vi "LESO_error.vi"(8 "error in":errorcluster, 11 "FT_Status":u32(ring) items=["FT_OK", "FT_INVALID_HANDLE", "FT_DEVICE_NOT_FOUND", "FT_DEVICE_NOT_OPENED", "FT_IO_ERROR", "FT_INSUFFICIENT_RESOURCES", "FT_INVALID_PARAMETER", "FT_INVALID_BAUD_RATE", "FT_DEVICE_NOT_OPENED_FOR_ERASE", "FT_DEVICE_NOT_OPENED_FOR_WRITE", "FT_FAILED_TO_WRITE_DEVICE", "FT_EEPROM_READ_FAILED", "FT_EEPROM_WRITE_FAILED", "FT_EEPROM_ERASE_FAILED", "FT_EEPROM_NOT_PRESENT", "FT_EEPROM_NOT_PROGRAMMED", "FT_INVALID_ARGS", "FT_NOT_SUPPORTED", "FT_OTHER_ERROR"]) -> (0 "error out":errorcluster)   [LabVIEW 2012]
doc: "Преобразует <B>FT_Status</B> в ошибку. Если <B>FT_Status</B> не равен <B>FT_OK</B>, то добавляет ошибку в кластер ошибок. В описании ошибки будет имя текущего ВП и <B>FT_Status</B>."
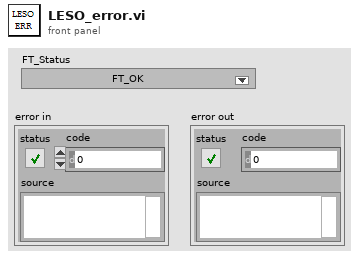
[diagram p1: front panel]
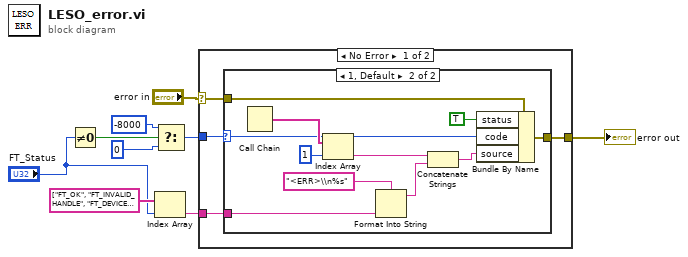
[diagram p0: block diagram]
diagram:
  n1 = Not Equal To 0?(x="FT_Status") -> (x != 0?=w8:bool)
  n2 = Index Array(array=string[] ["FT_OK", "FT_INVALID_HANDLE", "FT_DEVICE_NOT_FOUND", "FT_DEVICE_NOT_OPENED", "FT_IO_ERROR", "FT_INSUFFICIENT_RESOURCES", "FT_INVALID_PARAMETER", "FT_INVALID_BAUD_RATE", "FT_DEVICE_NOT_OPENED_FOR_ERASE", "FT_DEVICE_NOT_OPENED_FOR_WRITE", "FT_FAILED_TO_WRITE_DEVICE", "FT_EEPROM_READ_FAILED", "FT_EEPROM_WRITE_FAILED", "FT_EEPROM_ERASE_FAILED", "FT_EEPROM_NOT_PRESENT", "FT_EEPROM_NOT_PROGRAMMED", "FT_INVALID_ARGS", "FT_NOT_SUPPORTED", "FT_OTHER_ERROR"] ("Status"), index="FT_Status") -> (element=w6:string)
  n3 = Select(t=-8000 ("error code (0)"), s=w8, f=0) -> (s? t:f=w3:i32)
  n4 = case shown="No Error" "error in" {
    selector: "error in" -> [w10 w26]
    tunnel: [w13 w26] -> w2
    tunnel: w3 -> [w11 _]
    tunnel: w6 -> [w12 _]
    frame No Error {
      n5 = case shown="1, Default" w11 {
        selector: w11 -> [_ w16]
        tunnel: [w14 w25] -> w13
        tunnel: w12 -> [_ w24]
        tunnel: w10 -> [w14 w15]
        frame 0 {
          # "Статус равен нулю, ошибки нет."
        }
        frame 1, Default {
          n6 = Call Chain() -> (call chain=w21:string[])
          n7 = Index Array(array=w21, index=1) -> (element=w18:string)
          n8 = Format Into String(format string="<ERR>\\n%s", w24) -> (resulting string=w19:string)  [unwired: 2 in, 1 out]
          n9 = Concatenate Strings(w18, w19) -> (w23:string)
          n10 = Bundle By Name(cluster=w15, "status"=TRUE, "code"=w16, "source"=w23) -> (w25:errorcluster)
        }
      }
    }
    frame Error {
      # "На входе уже ошибка,\nпропускаем ее без изменений на выход"
    }
  }
  "error out" <- w2
